vi "Copy Libs.vi"() -> ()   [LabVIEW 2019]
panel:
  in  "vendordeps list":path[](array[path])=[path "../WPILib-Wrapper/vendordeps/LabVIEW_WPILib_Extensions.json"]
  in  "output":path=path "./lib"
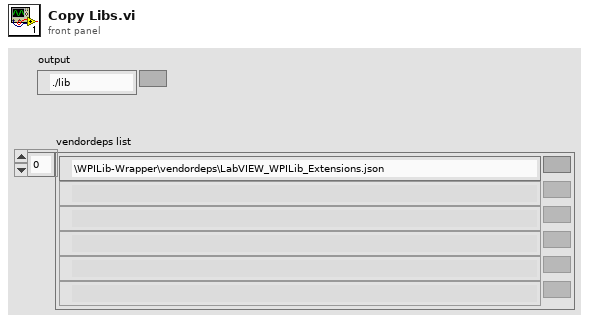
[diagram p1: front panel]
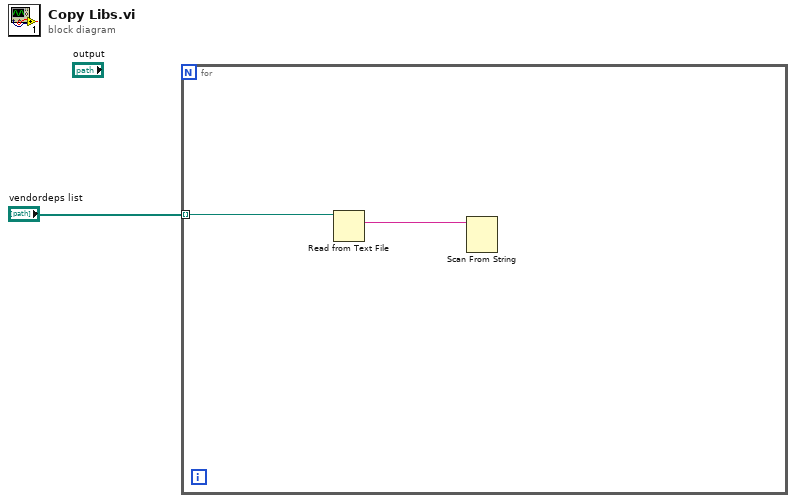
[diagram p0: block diagram]
diagram:
  n1 = for {
    tunnel: "vendordeps list" -> [w3] mode=indexing
    n2 = Read from Text File(file (use dialog)=w3) -> (text=w2:string)  [unwired: 3 in, 3 out]
    n3 = Scan From String(input string=w2) -> ()  [unwired: 5 in, 3 out]
  }
